vi "AI Index Element.vi"(9 "AI Index Element":i32[](array[numeric]), 11 "Write/Read":enum16{"Write", "Read"}(ring)=enum."Read") -> (1 "Ai Index Element":i32[](array[numeric]))   [LabVIEW 2020]
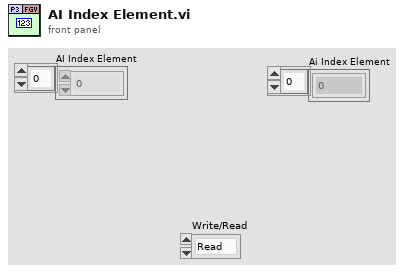
[diagram p1: front panel]
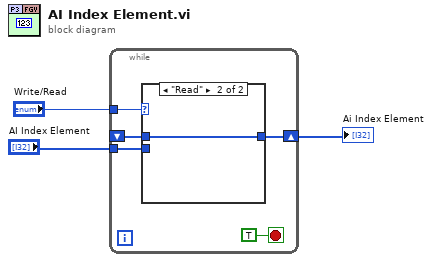
[diagram p0: block diagram]
diagram:
  n1 = while {
    tunnel: "Write/Read" -> [w7]
    shift-right: [w6] -> w1
    shift-left: _ -> [w5]
    tunnel: "AI Index Element" -> [w4]
    stop <- TRUE stop-if-true
    n2 = case shown="\"Read\"" w7 {
      tunnel: [w9 w10] -> w6
      tunnel: w5 -> [_ w10]
      tunnel: w4 -> [w9 _]
      frame "Write" {
      }
      frame "Read" {
      }
    }
  }
  "Ai Index Element" <- w1
